vi "fft_subvi.vi"(10 "Fs":i32=2000, 11 "Array":dbl[](array[numeric])) -> (3 "Waveform Graph":waveform(dbl)(graph))   [LabVIEW 2016]
doc: "FFT transform. Analysis spectrum of signal"
uses:
  <vilib>/Analysis/2dsp.llb/Real FFT.vi
  <vilib>/Analysis/NI_AALPro.lvlib
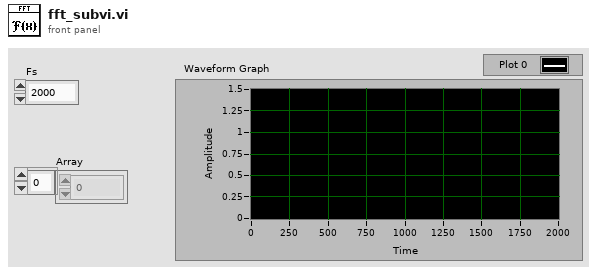
[diagram p1: front panel]
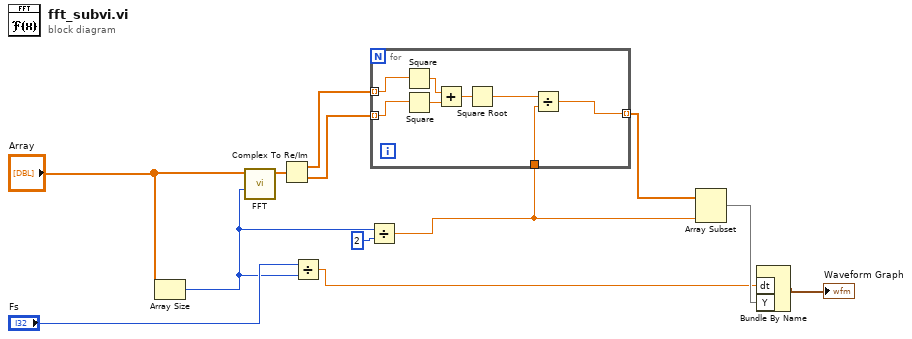
[diagram p0: block diagram]
diagram:
  n1 = Array Size(array="Array") -> (size(s)=w3:i32)
  n2 = call-poly <vilib>:"FFT.vi"("FFT size"=w3, "X"="Array") -> ("FFT {X}"=w11:cdb[])  [unwired: 8 in, 1 out]
  n3 = Complex To Re/Im(x + iy=w11) -> (x=w10:dbl[], y=w9:dbl[])
  n4 = Divide(x="Fs", y=w3) -> (x/y=w2:dbl)
  n5 = Divide(x=w3, y=2) -> (x/y=w1:dbl)
  n6 = for {
    tunnel: w10 -> [w18] mode=indexing
    tunnel: w9 -> [w17] mode=indexing
    tunnel: [w14] -> w8 mode=indexing
    tunnel: w1 -> [w13]
    n7 = Square(x=w18) -> (x^2=w16:dbl)
    n8 = Square(x=w17) -> (x^2=w19:dbl)
    n9 = Add(x=w16, y=w19) -> (x+y=w20:dbl)
    n10 = Square Root(x=w20) -> (sqrt(x)=w15:dbl)
    n11 = Divide(x=w15, y=w13) -> (x/y=w14:dbl)
  }
  n12 = Array Subset(array=w8, length=w1) -> (w6:dbl[])  [unwired: 1 in]
  n13 = Bundle By Name("dt"=w2, "Y"=w6) -> (→"Waveform Graph":waveform(dbl))  [unwired: 1 in]
